vi "2ItemVectorAdd.vi"(10 "Vector 2":cluster{dbl, dbl}, 11 "Vector 1":cluster{dbl, dbl}) -> (3 "Resultant Vector":cluster{dbl, dbl})   [LabVIEW 2013]
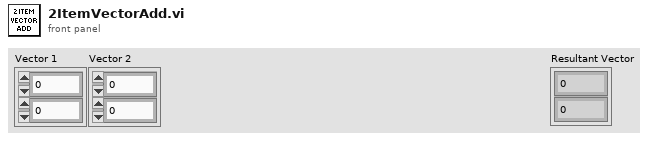
[diagram p1: front panel]
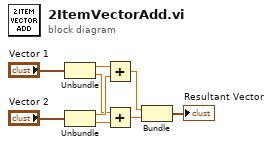
[diagram p0: block diagram]
diagram:
  n1 = Unbundle("Vector 1") -> (w7:dbl, w4:dbl)
  n2 = Unbundle("Vector 2") -> (w6:dbl, w3:dbl)
  n3 = Add(x=w7, y=w6) -> (x+y=w5:dbl)
  n4 = Add(x=w4, y=w3) -> (x+y=w2:dbl)
  n5 = Bundle(w5, w2) -> (→"Resultant Vector":cluster{dbl, dbl})  [unwired: 1 in]
